vi "Test Logger Normal.vi"   [LabVIEW 2020]
uses:
  Normal Log/Normal Log/Normal Log.lvclass
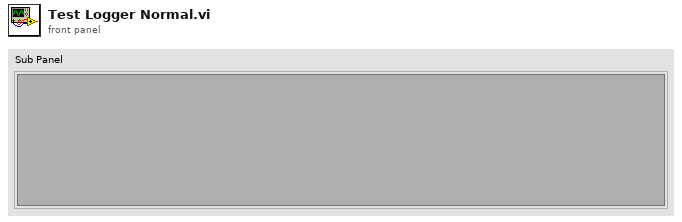
[diagram p1: front panel]
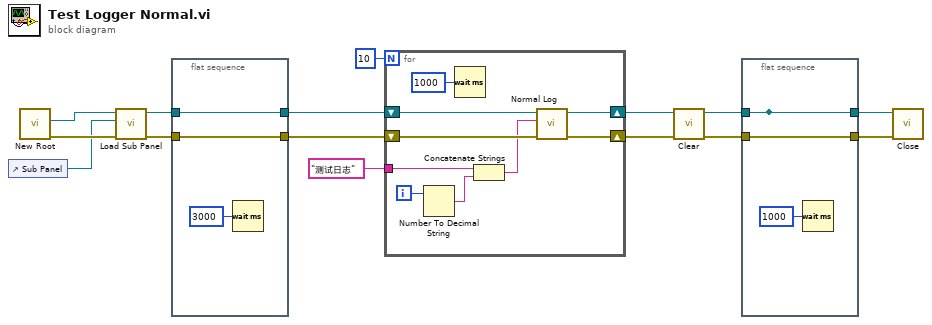
[diagram p0: block diagram]
diagram:
  n1 = control-ref of="Sub Panel"() -> (w7:refnum<vi>)
  n2 = call "New Root.vi"() -> ("error out"=w11:errorcluster, "normal log"=w8:refnum<class "Normal Log.lvclass">)  [unwired: 10 in]
  n3 = call-dynamic "Load Sub Panel.vi"("error in (no error)"=w11, "sub panel"=w7, "Normal Log in"=w8) -> ("error out"=w10:errorcluster, "Normal Log out"=w9:refnum<class "Normal Log.lvclass">)  [unwired: 7 in]
  n4 = flat-sequence {
    tunnel: w9 -> [w17]
    tunnel: w10 -> [w16]
    tunnel: [w17] -> w13
    tunnel: [w16] -> w12
    frame #0 {
      n5 = Wait (ms)(milliseconds to wait=u32 3000) -> ()  [unwired: 1 out]
    }
  }
  n6 = for {
    N: 10 -> [_]
    shift-right: [w25] -> w4
    shift-left: w13 -> [w27]
    shift-right: [w24] -> w5
    shift-left: w12 -> [w26]
    tunnel: "测试日志" -> [w22]
    i -> [w20]
    n7 = Number To Decimal String(number=w20) -> (decimal integer string=w19:string)  [unwired: 1 in]
    n8 = Wait (ms)(milliseconds to wait=u32 1000) -> ()  [unwired: 1 out]
    n9 = Concatenate Strings(w22, w19) -> (w21:string)
    n10 = call-dynamic "Normal Log.vi"("error in (no error)"=w26, "log"=w21, "Normal Log in"=w27) -> ("error out"=w24:errorcluster, "Normal Log out"=w25:refnum<class "Normal Log.lvclass">)  [unwired: 7 in]
  }
  n11 = call-dynamic "Clear.vi"("error in (no error)"=w5, "Normal Log in"=w4) -> ("error out"=w6:errorcluster, "Normal Log out"=w3:refnum<class "Normal Log.lvclass">)  [unwired: 8 in]
  n12 = flat-sequence {
    tunnel: w3 -> [w28]
    tunnel: w6 -> [w29]
    tunnel: [w28] -> _
    tunnel: [w29] -> w2
    tunnel: [w28] -> w1
    frame #0 {
      n13 = Wait (ms)(milliseconds to wait=u32 1000) -> ()  [unwired: 1 out]
    }
  }
  n14 = call-dynamic "Close.vi"("error in (no error)"=w2, "Normal Log in"=w1) -> ()  [unwired: 9 in, 1 out]
